vi "OSORIO_JHOEL_PROYECTO_PUNTOS.vi"() -> ()   [LabVIEW 2026]
uses:
  <vilib>/MakerHub/LINX/Public/Peripherals/Analog/Analog Read 1 Chan.vi
  <vilib>/MakerHub/LINX/Public/Peripherals/Analog/Analog Read N Chans.vi
  <vilib>/MakerHub/LINX/Private/Local IO/LinxAnalogRead.vi
  <vilib>/MakerHub/LINX/Public/Utilities/Check Channel.vi
  <vilib>/MakerHub/LINX/Public/Utilities/Open Serial.vi
  <vilib>/MakerHub/LINX/Private/Utilties/Generate Error.vi
  <vilib>/express/express arith-compare/Formula/XNode/ExpressFormulaBlockNode.xnode
  <vilib>/MakerHub/LINX/LMH-LINX.lvlib
panel:
  out "%LUZ":dbl
  out "%TANQUE":dbl
  out "TARDE":bool
  out "MAÑANA":bool
  out "NOCHE":bool
  out "TANQUE VACIO !!":bool
  out ">33%-67%<":bool
  out "<33%":bool
  out ">67%":bool
  out "LUZ":dbl(slide) scale=0.0..100.0
  out "TANQUE":dbl(slide) scale=0.0..100.0
  in  "Serial Port":refnum<visa-resource-name>="N/A"
  in  "STOP":bool
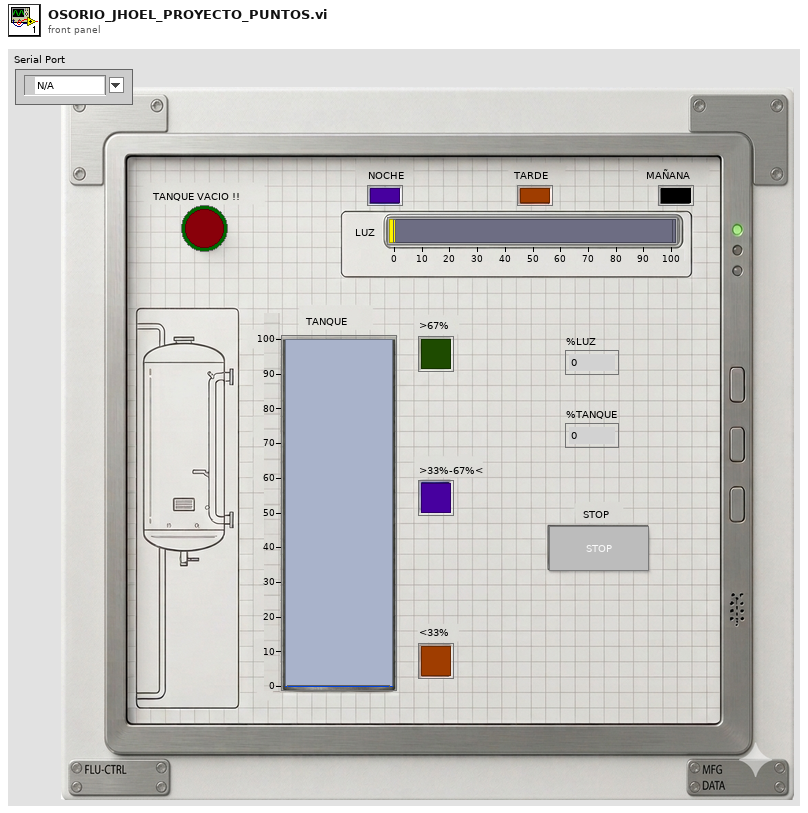
[diagram p1: front panel]
types:
  T1 = typedef "LMH-LINX.lvlib/LINX Ref.ctl" = cluster{"IO":T2, "Interface":T3, "LINX Device Config":T4}
  T2 = typedef "LMH-LINX.lvlib/Platform.ctl" = enum16{"Remote", "Local"}
  T3 = typedef "LMH-LINX.lvlib/Interface.ctl" = enum16{"Serial", "TCP"}
  T4 = typedef "LMH-LINX.lvlib/Device.lvlib/LINX Device Config.ctl" = cluster{"Interface":T3, "COM Port":refnum<visa-resource-name>, "TCP Configuration":T5, "Device Family":u8, "Device ID":u8, "Device Name":string, "TCP Ref":refnum<k5>, "Channels":T6}
  T5 = typedef "LMH-LINX.lvlib/Device.lvlib/TCP Config.ctl" = cluster{"IP Address":string, "Port":u16}
  T6 = typedef "LMH-LINX.lvlib/Channels.ctl" = cluster{"DI":u8[], "DO":u8[], "AI":u8[], "AO":u8[], "PWM":u8[], "QE":u8[], "UART":u8[], "I2C 2":u8[], "SPI":u8[], "CAN":u8[], "Servo":u8[], "AI Ref (V)":dbl, "AI Resolution (Bits)":u8, "AO Ref (V)":dbl, "AO Resolution (Bits)":u8}
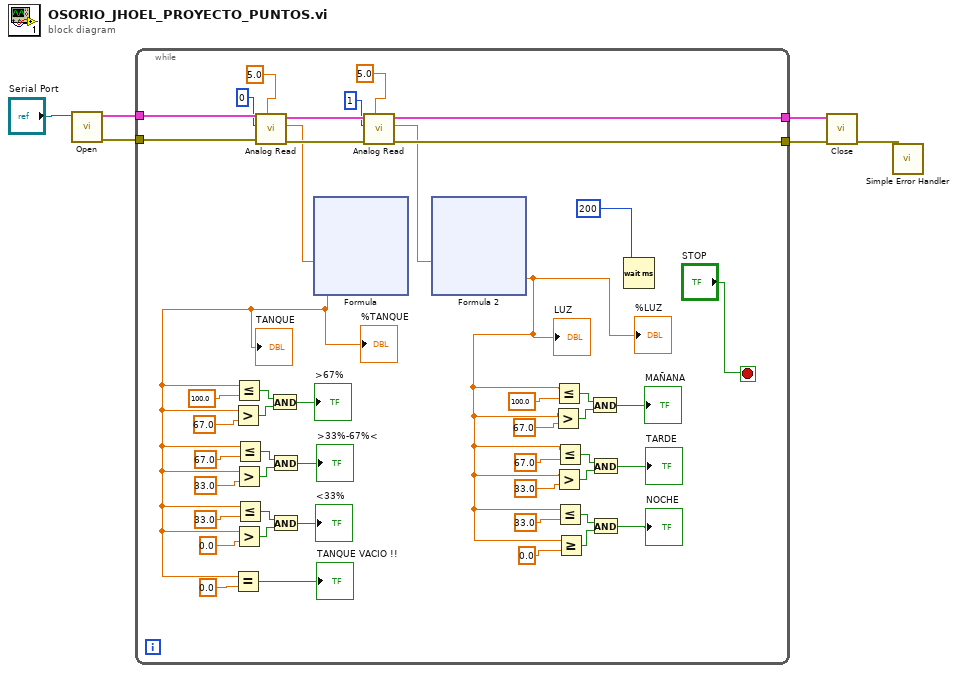
[diagram p0: block diagram]
diagram:
  n1 = call-poly <vilib>:"Open.vi"("Serial Port"="Serial Port") -> ("Error Out"=w3:errorcluster, "LINX Resource"=w4:T1)  [unwired: 8 in, 1 out]
  n2 = while {
    tunnel: w4 -> [w54]
    tunnel: w3 -> [w53]
    tunnel: [w43] -> w2
    tunnel: [w44] -> w1
    stop <- "STOP" stop-if-true
    n3 = call-poly <vilib>:"Analog Read.vi"("Analog Ref Override (V)"=5.0, "Error In"=w53, "Analog Channel"=0, "LINX Resource"=w54) -> ("Error Out"=w51:errorcluster, "Voltage"=w42:dbl, "LINX Resource"=w52:T1)  [unwired: 4 in, 1 out]
    n4 = xnode "Formula"("X1"=w42) -> ("Result"=w8:dbl)  [unwired: 1 in, 1 out]
    "TANQUE" <- w8
    "%TANQUE" <- w8
    n5 = Greater?(x=w8, y=67.0) -> (0:w39:bool)
    n6 = Equal?(x=w8, y=0.0) -> (x = y?=→"TANQUE VACIO !!":bool)
    n7 = Less Or Equal?(x=w8, y=100.0) -> (x <= y?=w37:bool)
    n8 = Greater?(x=w8, y=33.0) -> (0:w34:bool)
    n9 = Greater?(x=w8, y=0.0) -> (0:w30:bool)
    n10 = Less Or Equal?(x=w8, y=67.0) -> (x <= y?=w33:bool)
    n11 = Less Or Equal?(x=w8, y=33.0) -> (x <= y?=w29:bool)
    n12 = And(x=w37, y=w39) -> (x .and. y?=→">67%":bool)
    n13 = And(x=w33, y=w34) -> (x .and. y?=→">33%-67%<":bool)
    n14 = And(x=w29, y=w30) -> (x .and. y?=→"<33%":bool)
    n15 = call-poly <vilib>:"Analog Read.vi"("Analog Ref Override (V)"=5.0, "Error In"=w51, "Analog Channel"=1, "LINX Resource"=w52) -> ("Error Out"=w43:errorcluster, "Voltage"=w41:dbl, "LINX Resource"=w44:T1)  [unwired: 4 in, 1 out]
    n16 = xnode "Formula 2"("X1"=w41) -> ("Result"=w7:dbl)  [unwired: 1 in, 1 out]
    "LUZ" <- w7
    "%LUZ" <- w7
    n17 = Greater?(x=w7, y=67.0) -> (0:w22:bool)
    n18 = Less Or Equal?(x=w7, y=100.0) -> (x <= y?=w21:bool)
    n19 = Greater?(x=w7, y=33.0) -> (0:w18:bool)
    n20 = Less Or Equal?(x=w7, y=67.0) -> (x <= y?=w17:bool)
    n21 = Less Or Equal?(x=w7, y=33.0) -> (x <= y?=w15:bool)
    n22 = Greater Or Equal?(x=w7, y=0.0) -> (x >= y?=w9:bool)
    n23 = And(x=w21, y=w22) -> (x .and. y?=→"MAÑANA":bool)
    n24 = And(x=w17, y=w18) -> (x .and. y?=→"TARDE":bool)
    n25 = And(x=w15, y=w9) -> (x .and. y?=→"NOCHE":bool)
    n26 = Wait (ms)(milliseconds to wait=u32 200 ("millisecond timer value")) -> ()  [unwired: 1 out]
  }
  n27 = call <vilib>:"Close.vi"("Error In"=w2, "LINX Resource"=w1) -> ("Error Out"=w5:errorcluster)  [unwired: 9 in]
  n28 = call <vilib>:"Simple Error Handler.vi"("error in (no error)"=w5) -> ()  [unwired: 4 in, 5 out]
